vi "Ammeter Shutdown (Poly).vi"   [LabVIEW 2016, in "Hall Effect Library.lvlib"]
uses:
  Hall Effect Library.lvlib
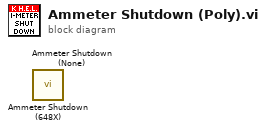
[diagram p0: block diagram]
diagram:
  n1 = call "Ammeter Shutdown (648X).vi"() -> ()  [unwired: 10 in, 2 out]
  n2 = call "Ammeter Shutdown (None).vi"() -> ()  [unwired: 10 in, 2 out]
